vi "Pre-order Visit.vi"(8 "error in (no error)":errorcluster, 9 "User Data In":variant, 10 "Visitor VI":T1, 11 "AST in":refnum<class "AST.lvclass">) -> (0 "error out":errorcluster, 1 "User Data":variant, 3 "AST out":refnum<class "AST.lvclass">)   [LabVIEW 2020, in "PicoG-ParserLexer.lvlib" / "AST.lvclass"]
uses:
  AST.lvclass
  Visitor VI.ctl
  Node/Node.lvclass
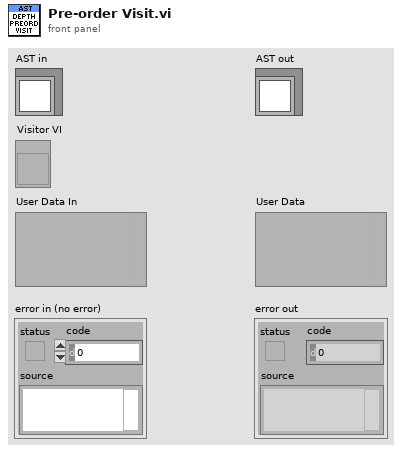
[diagram p1: front panel]
types:
  T1 = typedef "PicoG-ParserLexer.lvlib/AST.lvclass/Visitor VI.ctl" = refnum<vi>
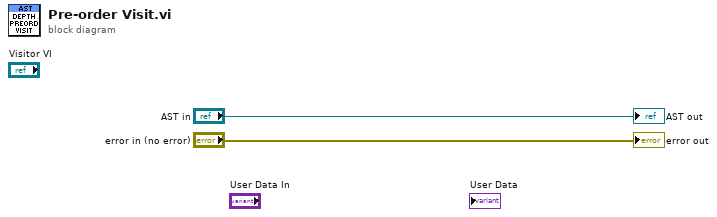
[diagram p0: block diagram]
diagram:
  "error out" <- "error in (no error)"
  "AST out" <- "AST in"
